vi "Example Edit.vi"() -> ()   [LabVIEW 2019]
uses:
  lib/JSON Action.ctl
  248ad171-fbf9-4f2e-ab24-158922efdba7.vi
  lib/JSON Edit.vi
  lib/labview_json.lvlib
panel:
  out "Value out":cluster{"powers":string[], "age":i32}
  in  "Action":T1
  in  "Value in":cluster{"powers":string[], "age":i32}={"powers"=["earth", "fire", "wind", "water"], "age"=89}
  out "JSON out":string
  out "Exists?":bool
  out "Error":errorcluster
  in  "JSON in":string="{\n  \"squadName\": \"Super hero squad\",\n  \"homeTown\": \"Metro City\",\n  \"formed\": 2016,\n  \"secretBase\": \"Super tower\",\n  \"active\": true,\n  \"members\": [\n    {\n      \"name\": \"Molecule Man\",\n      \"age\": 29,\n      \"secretIdentity\": \"Dan Jukes\",\n      \"powers\": [\n        \"Radiation resistance\",\n        \"Turning tiny\",\n        \"Radiation blast\"\n      ]\n    },\n    {\n      \"name\": \"Madame Uppercut\",\n      \"age\": 39,\n      \"secretIdentity\": \"Jane Wilson\",\n      \"powers\": [\n        \"Million tonne punch\",\n        \"Damage resistance\",\n        \"Superhuman reflexes\"\n      ]\n    },\n    {\n      \"name\": \"Eternal Flame\",\n      \"age\": 1000000,\n      \"secretIdentity\": \"Unknown\",\n      \"powers\": [\n        \"Immortality\",\n        \"Heat Immunity\",\n        \"Inferno\",\n        \"Teleportation\",\n        \"Interdimensional travel\"\n      ]\n    }\n  ]\n}"
  in  "Root Path":string[](array[string])=["members", "0"]
  # "1."
  # "2."
  # "6."
  # "The root path is the nested \nobject key or array index\nto the element you want\nto get or set.\nObjects = Key\nArrays = Index"
  # "3."
  # "7."
  # "4."
  # "5."
  # "Instructions:\nFrom the JSON string (1.) select the Action (2.) as:\n    Get or Create = Reads or creates the value elements\n    Get = Only read the value elements, do not create\n    Set = Write or create the value elements\nspecify the Root Path (3.) to the nested element to where\n    Array Index : INT = Integer of the array index where 0 is the first index in the array (e.g. 1)\n    Object Key : STR = String object key name (e.g. \"age\")"
  # "Instructions (cont.):\nSpecify the LabVIEW Value (4.) to unflatten the JSON string into, if the element\ndoes not exist, this uses the default Value inputs. \nDepending on the Action, the Value out (5.) is the parsed LabVIEW data and the\nJSON out (6.) is the JSON string modified. \nExists? (7.) returns true if all elements exist for the object."
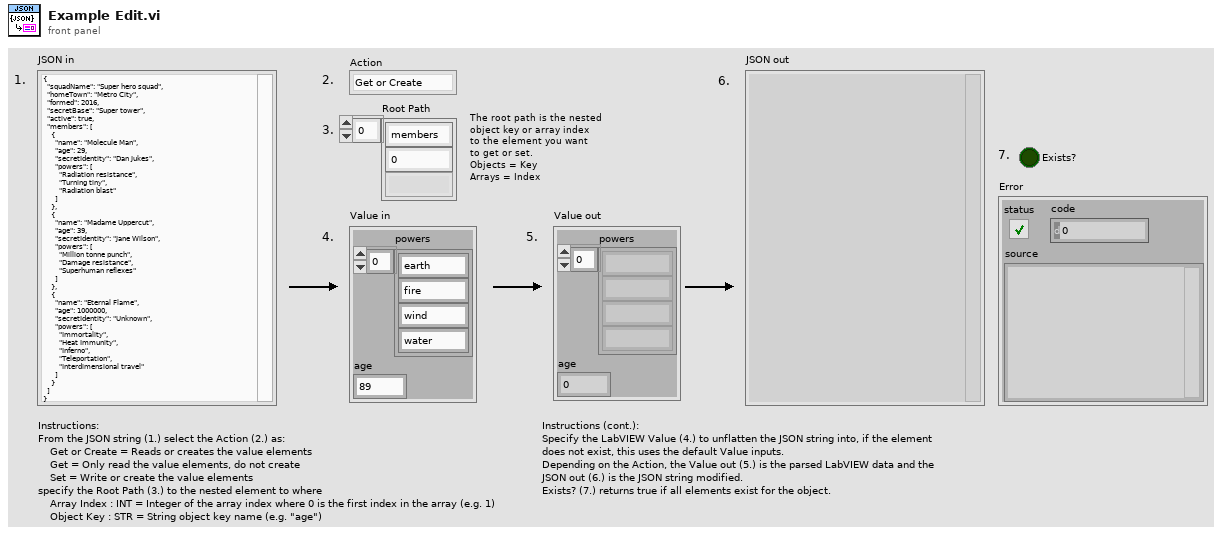
[diagram p1: front panel]
types:
  T1 = typedef "labview_json.lvlib/JSON Action.ctl" = enum8{"Get or Create", "Get", "Set"}
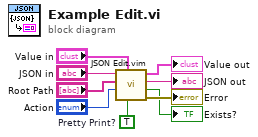
[diagram p0: block diagram]
diagram:
  w9 = TRUE  # Pretty Print?
  n1 = call "JSON Edit.vim"("Pretty Print? (F)"=w9, "Variant in"="Value in", "Action (Get or Create)"="Action", "Root Path ([]=Root)"="Root Path", "JSON in"="JSON in") -> ("error out"=→"Error":errorcluster, "Exists?"=→"Exists?":bool, "JSON out"=→"JSON out":string, "Variant out"=→"Value out":cluster{"powers":string[], "age":i32})  [unwired: 3 in]
